vi "CT.vi"(1 "Ctl Refnum 2":refnum<vi>, 2 "Ctl Refnum":refnum<vi>, 7 "测试时长":dbl, 8 "error in (no error)":errorcluster caption="错误输入（无错误）", 9 "客户仪器地址":refnum<visa-resource-name>="USB0::0x0471::0x2826::QF71600867::INSTR", 10 "测试频率":dbl=100000.0, 11 "Cluster 2":cluster{"文本数据路径：":path, "表格数据路径： ":path}={"文本数据路径："=path "C:/Users/shipeng/Desktop/LT Dielectric measurement", "表格数据路径： "=path "C:/Users/shipeng/Desktop/LT Dielectric measurement"}) -> (0 "错误输出":cluster{"状态":bool, "代码":i32, "源":string})   [LabVIEW 2017]
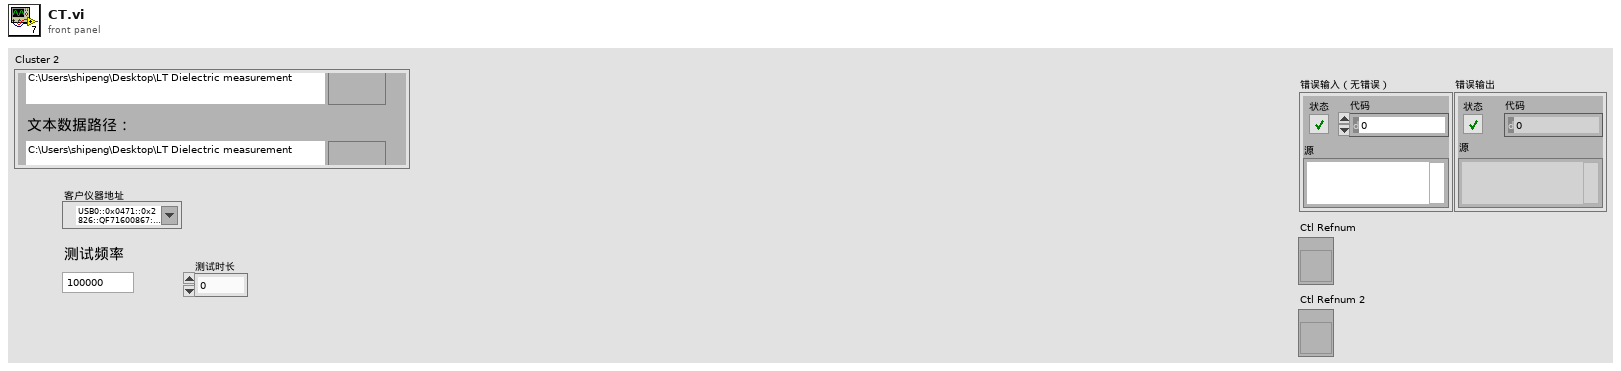
[diagram p1: front panel]
types:
  T1 = enum16{"open", "replace", "create", "open or create", "replace or create", "replace or create with confirmation"}
  T2 = cluster{"VISA resource name 2":refnum<visa-resource-name>, "refnum out":refnum<file>, "测试频率":dbl, "error out":errorcluster}
  T3 = cluster{"Array":string[][], "error out":errorcluster}
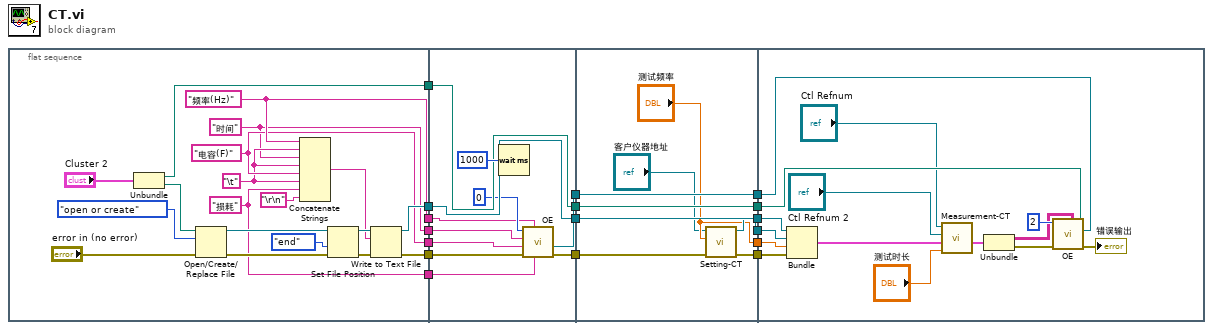
[diagram p0: block diagram]
diagram:
  n1 = flat-sequence {
    tunnel: [w29] -> w17
    tunnel: [w28] -> w16
    tunnel: [w26] -> w13
    tunnel: [w25] -> w12
    tunnel: [w24] -> w11
    tunnel: [w20] -> w8
    tunnel: [w19] -> w7
    tunnel: w17 -> [w46]
    tunnel: [w46] -> w15
    tunnel: [w37] -> w14
    tunnel: w16 -> [w39]
    tunnel: w13 -> [w43]
    tunnel: w12 -> [w40]
    tunnel: w11 -> [w41]
    tunnel: [w38] -> w10
    tunnel: [w45] -> w9
    tunnel: w8 -> [w45]
    tunnel: w7 -> [w42]
    tunnel: w15 -> [w55]
    tunnel: [w55] -> w6
    tunnel: w14 -> [w51]
    tunnel: [w52] -> w5
    tunnel: [w54] -> w4
    tunnel: w10 -> [w54]
    tunnel: ["测试频率"] -> w3
    tunnel: [w53] -> w2
    tunnel: w9 -> [w53]
    tunnel: [w50] -> w1
    tunnel: w6 -> [w69]
    tunnel: w5 -> [w70]
    tunnel: w4 -> [w67]
    tunnel: w3 -> [w68]
    tunnel: w2 -> [w66]
    tunnel: w1 -> [w57]
    frame #0 {
      w19 = "时间" ("字符串")
      w25 = "损耗" ("字符串")
      w24 = "电容(F)" ("字符串")
      w23 = "\t"
      w26 = "频率(Hz)" ("字符串")
      n2 = Unbundle("Cluster 2") -> ("文本数据路径："=w20:path, "表格数据路径："=w21:path)
      n3 = Open/Create/Replace File(file path (use dialog)=w21, error in="error in (no error)", operation (0:open)=T1."open or create" ("操作(0:open)")) -> (refnum out=w34:refnum<file>, error out=w31:errorcluster)  [unwired: 4 out]
      n4 = Concatenate Strings(w26, w23, w19, w23, w24, w23, w25, "\r\n") -> (w30:string)
      n5 = Set File Position(refnum=w34, from (0:start)=enum16{"start", "end", "current"}."end" ("自（0:起始）"), error in=w31) -> (refnum out=w35:refnum<file>, error out=w36:errorcluster)  [unwired: 1 out]
      n6 = Write to Text File(file (use dialog)=w35, text=w30, error in=w36) -> (refnum out=w29:refnum<file>, error out=w28:errorcluster)  [unwired: 2 out]
    }
    frame #1 {
      n7 = Wait (ms)(milliseconds to wait=u32 1000 ("等待时间（毫秒）")) -> ()  [unwired: 1 out]
      n8 = call "OE.vi"("String 4"=w40, "String"=w43, "error in (no error)"=w39, "String 3"=w41, "String 2"=w42, "Numeric"=0) -> ("error out"=w37:errorcluster, "report out"=w38:refnum<class "NI_report.lvclass">)  [unwired: 3 in, 1 out]
    }
    frame #2 {
      n9 = call "Setting-CT.vi"("error in (no error)"=w51, "number"="测试频率", "VISA resource name"="客户仪器地址") -> ("error out"=w52:errorcluster, "VISA resource name 2"=w50:refnum<visa-resource-name>)  [unwired: 7 in]
    }
    frame #3 {
      n10 = Bundle("VISA resource name 2"=w57, "refnum out"=w69, "测试频率"=w68, "error out"=w70) -> (w63:T2)  [unwired: 1 in]
      n11 = call "Measurement-CT.vi"("Numeric"="测试时长", "Cluster 2"=w63, "Ctl Refnum 2"="Ctl Refnum 2", "Ctl Refnum"="Ctl Refnum") -> ("Cluster"=w62:T3)  [unwired: 7 in]
      n12 = Unbundle(w62) -> ("Array"=w60:string[][], "error out"=w61:errorcluster)
      n13 = call "OE.vi"("report in"=w67, "表格数据路径："=w66, "Array"=w60, "error in (no error)"=w61, "Numeric"=2) -> ("error out"=→"错误输出":errorcluster)  [unwired: 4 in, 2 out]
    }
  }
